vi "Round.vi"(4 "place at this power of 10":i32, 7 "Number In":dbl format="%#_12f") -> (3 "Number Out":dbl format="%#_12g")   [LabVIEW 2023]
doc: "Round a number to a decimal place specified by its corresponding power of ten. Rounding 1234.567 to \"1\" (10^1) results in 1230.0. Rounding 1234.567 to \"-2\" (10^-2) results in 1234.57."
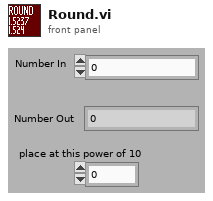
[diagram p1: front panel]
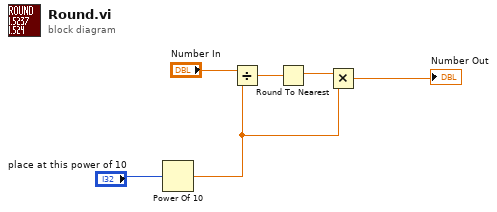
[diagram p0: block diagram]
diagram:
  n1 = Power Of 10(x="place at this power of 10") -> (10^x=w2:dbl)
  n2 = Divide(x="Number In", y=w2) -> (x/y=w4:dbl)
  n3 = Round To Nearest(number=w4) -> (nearest integer value=w3:dbl)
  n4 = Multiply(x=w3, y=w2) -> (x*y=→"Number Out":dbl)
